vi "Global Launch.vi"(8 "error in (no error)":errorcluster, 10 "App + Modules":T1[](array[typedef]), 11 "Global in":refnum<k1>) -> (0 "error out":errorcluster, 2 "App ID":i32, 3 "Global out":refnum<k1>)   [LabVIEW 2018, in "Shared.lvlib"]
uses:
  Shared.lvlib
  Controls/Global.ctl
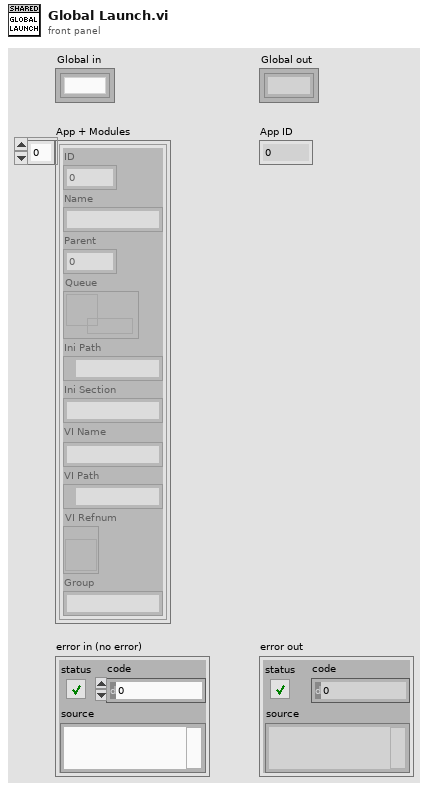
[diagram p1: front panel]
types:
  T1 = typedef "Shared.lvlib/Global.ctl" = cluster{"ID":i32, "Name":string, "Parent":i32, "Queue":refnum<queue>, "Ini Path":path, "Ini Section":string, "VI Name":string, "VI Path":path, "VI Refnum":refnum<vi>, "Group":string}
  T2 = enum32{"Invalid", "Standard", "Closed", "Hidden", "Minimized", "Maximized"}
  T3 = cluster{"ID":i32, "Name":string, "Parent":i32, "Queue":refnum<queue>, "Ini Path":path, "Ini Section":string, "VI Name":string, "VI Path":path, "VI Refnum":refnum<vi>, "Group":string}[]
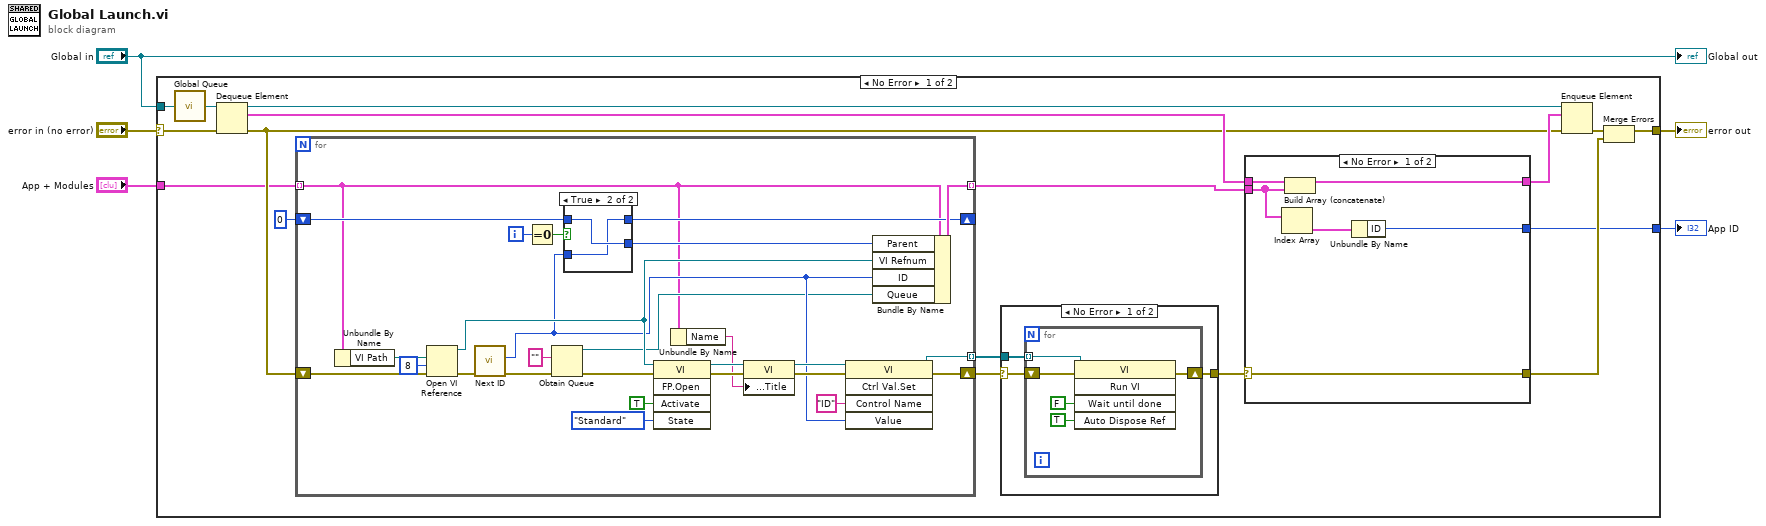
[diagram p0: block diagram]
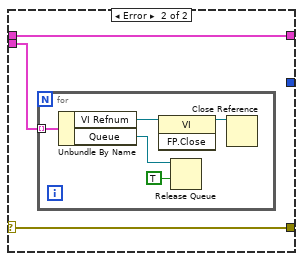
[diagram p4: hidden frame]
diagram:
  n1 = case shown="No Error" "error in (no error)" {
    selector: "error in (no error)" -> [w22 w76]
    tunnel: "Global in" -> [w21 _]
    tunnel: [w13 w76] -> w3
    tunnel: "App + Modules" -> [w7 _]
    tunnel: [w6 _] -> w1
    frame No Error {
      n2 = call "Global Queue.vi"("Global in"=w21) -> ("Global"=w20:refnum<queue>)
      n3 = Dequeue Element(queue=w20, error in (no error)=w22) -> (queue out=w18:refnum<queue>, element=w17:T3, error out=w10:errorcluster)  [unwired: 1 in, 1 out]
      n4 = for {
        tunnel: w7 -> [w36] mode=indexing
        tunnel: [w58] -> w15 mode=indexing
        shift-right: [w34] -> w14
        shift-left: w10 -> [w41]
        shift-right: [w53] -> _
        shift-left: 0 ("Next ID") -> [w55]
        tunnel: [w33] -> w8 mode=indexing
        i -> [w57]
        n5 = Unbundle By Name(w36) -> ("VI Path"=w35:path)
        n6 = Open VI Reference(vi path=w35, options=8, error in (no error)=w41) -> (vi reference=w39:refnum<vi>, error out=w44:errorcluster)  [unwired: 3 in]
        n7 = call "Next ID.vi"("error in (no error)"=w44) -> ("error out"=w42:errorcluster, "Next ID"=w38:i32)  [unwired: 8 in, 1 out]
        n8 = Equal To 0?(x=w57) -> (x = 0?=w56:bool)
        n9 = Obtain Queue(element data type="", error in (no error)=w42) -> (queue out=w37:refnum<queue>, error out=w40:errorcluster)  [unwired: 3 in, 1 out]
        n10 = case shown="True" w56 {
          tunnel: w38 -> [_ w60]
          tunnel: w55 -> [w59 w61]
          tunnel: [w59 w61] -> w54
          tunnel: [w59 w60] -> w53
          frame False {
          }
          frame True {
          }
        }
        n11 = invoke class="VI" method="FP.Open"(reference=w39, error in=w40, "Activate"=TRUE ("Activate?"), "State"=T2."Standard") -> (reference out=w48:refnum<vi>, error out=w52:errorcluster)  [unwired: 1 in, 3 out]
        n12 = Unbundle By Name(w36) -> ("Name"=w47:string)
        n13 = property class="VI"(reference=w48, error in=w52, "Front Panel.Title"=w47) -> (reference out=w46:refnum<vi>, error out=w49:errorcluster)
        n14 = invoke class="VI" method="Ctrl Val.Set"(reference=w46, error in=w49, "Control Name"="ID", "Value"=w38) -> (reference out=w33:refnum<vi>, error out=w34:errorcluster)  [unwired: 1 in, 3 out]
        n15 = Bundle By Name(cluster=w36, "Parent"=w54, "VI Refnum"=w39, "ID"=w38, "Queue"=w37) -> (w58:T1)
      }
      n16 = case shown="No Error" w14 {
        selector: w14 -> [w25 w31]
        tunnel: [w24 w31] -> w9
        tunnel: w8 -> [w23 _]
        frame No Error {
          n17 = for {
            shift-right: [w29] -> w24
            shift-left: w25 -> [w30]
            tunnel: w23 -> [w28] mode=indexing
            n18 = invoke class="VI" method="Run VI"(reference=w28, error in=w30, "Wait until done"=FALSE ("Wait Until Done"), "Auto Dispose Ref"=TRUE ("Auto Dispose Reference")) -> (error out=w29:errorcluster)  [unwired: 1 in, 4 out]
          }
        }
        frame Error {
        }
      }
      n19 = case shown="No Error" w9 {
        selector: w9 -> [w65 w70]
        tunnel: w17 -> [w67 w69]
        tunnel: [w66 w69] -> w16
        tunnel: w15 -> [w64 w68]
        tunnel: [w65 w70] -> w12
        tunnel: [w62 _] -> w6
        frame No Error {
          n20 = Index Array(array=w64) -> (element=w63:T1)  [unwired: 1 in]
          n21 = Build Array (concatenate)(w67, w64) -> (w66:T1[])
          n22 = Unbundle By Name(w63) -> ("ID"=w62:i32)
        }
        frame Error {
          n23 = for {
            tunnel: w68 -> [w75] mode=indexing
            n24 = Unbundle By Name(w75) -> ("VI Refnum"=w74:refnum<vi>, "Queue"=w72:refnum<queue>)
            n25 = invoke class="VI" method="FP.Close"(reference=w74) -> (reference out=w73:refnum<vi>)  [unwired: 2 in, 2 out]
            n26 = Release Queue(queue=w72, force destroy? (F)=TRUE) -> ()  [unwired: 1 in, 3 out]
            n27 = Close Reference(reference=w73) -> ()  [unwired: 1 in, 1 out]
          }
        }
      }
      n28 = Enqueue Element(queue=w18, element=w16, error in (no error)=w10) -> (error out=w19:errorcluster)  [unwired: 1 in, 2 out]
      n29 = Merge Errors(w19, w12) -> (w13:errorcluster)
    }
    frame Error {
    }
  }
  "error out" <- w3
  "App ID" <- w1
  "Global out" <- "Global in"
